vi "FTW-SEQ-GetNextStep.vi"(8 "error in":errorcluster, 10 "Jobs Performed":i32, 11 "FTW Job Sequencer":refnum<class "FTW-JobSequencer.lvclass">) -> (0 "error out":errorcluster, 1 "Job Data":string, 2 "Current Job":string, 3 "FTW Job Sequencer out":refnum<class "FTW-JobSequencer.lvclass">)   [LabVIEW 2013, in "FTW-Actor.lvlib" / "FTW-JobSequencer.lvclass"]
uses:
  FTW-JobSequencer.lvclass
  FTW-JobSequencer.lvclass/FTW-JobSequencer.ctl
panel:
  # "Inputs"
  # "Outputs"
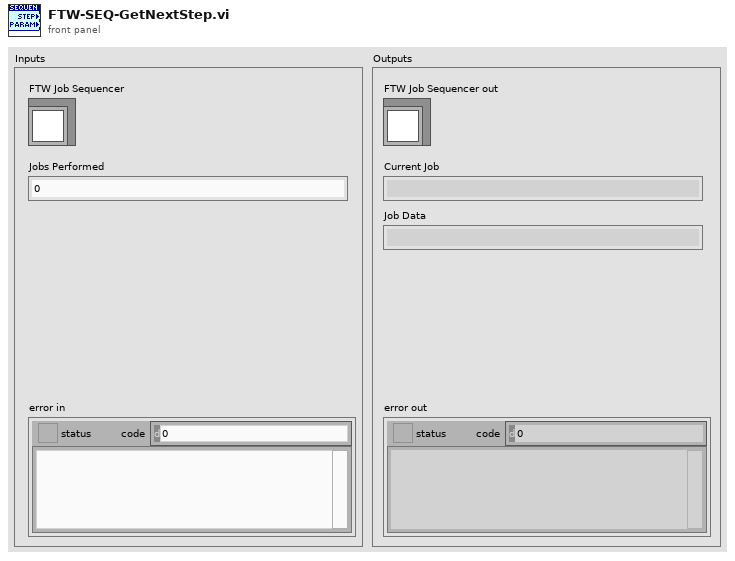
[diagram p1: front panel]
types:
  T1 = typedef "FTW-ERR-ExceptionType.ctl" = enum16{"No Error", "Error", "Warning"}
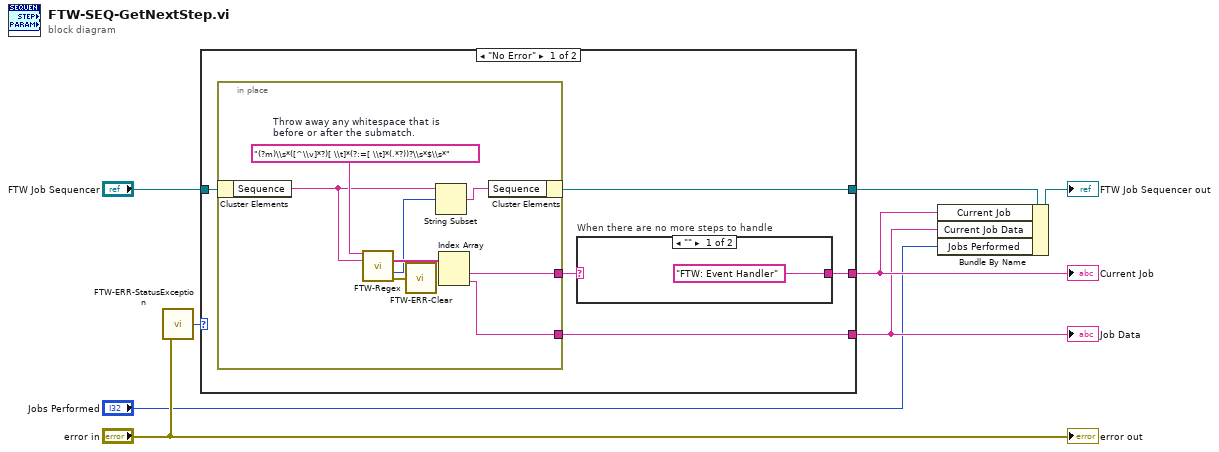
[diagram p0: block diagram]
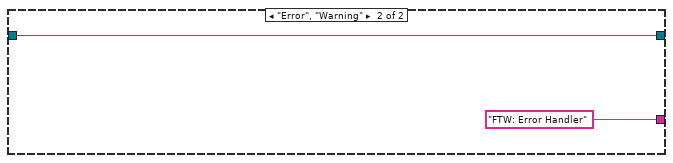
[diagram p3: hidden frame]
diagram:
  n1 = call "FTW-ERR-StatusException.vi"("error to check"="error in") -> ("Exception"=w6:T1)
  n2 = case shown="\"No Error\"" w6 {
    tunnel: "FTW Job Sequencer" -> [w10 w25]
    tunnel: [w12 "FTW: Error Handler" ("submatch 1")] -> w3
    tunnel: [w9 w25] -> w7
    tunnel: [w11 _] -> w2
    frame "No Error" {
      n3 = in-place {
        in-place-border: [w19] -> w13
        in-place-border: [w18] -> w11
        w21 = "(?m)\\s*([^\\v]*?)[ \\t]*(?:=[ \\t]*(.*?))?\\s*$\\s*"  # Throw away any whitespace that is before or after the submatch.
        n4 = in-place-cluster #1(w10) -> ("Sequence"=w17:string)
        n5 = call "FTW-Regex.vi"("Regular Expression"=w21, "Input String"=w17) -> ("Submatches"=w20:string[], "Offset after Match"=w16:i32, "error out"=w14:errorcluster)  [unwired: 9 in, 2 out]
        n6 = call "FTW-ERR-Clear.vi"("error to snuff"=w14) -> ()  [unwired: 1 out]
        n7 = String Subset(string=w17, offset (0)=w16) -> (substring=w15:string)  [unwired: 1 in]
        n8 = Index Array(array=w20) -> (element #1=w19:string, element #2=w18:string)  [unwired: 2 in]
        n9 = in-place-cluster #1("Sequence"=w15) -> (w9:refnum<class "FTW-JobSequencer.lvclass">)
      }
      n10 = case "When there are no more steps to handle" shown="\"\"" w13 {
        selector: w13 -> [_ w23]
        tunnel: ["FTW: Event Handler" w23] -> w12
        frame "" {
        }
        frame Default {
        }
      }
    }
    frame "Error", "Warning" {
    }
  }
  "Current Job" <- w3
  "Job Data" <- w2
  n11 = Bundle By Name(cluster=w7, "Current Job"=w3, "Current Job Data"=w2, "Jobs Performed"="Jobs Performed") -> (→"FTW Job Sequencer out":refnum<class "FTW-JobSequencer.lvclass">)
  "error out" <- "error in"
